vi "Engine Dynamics.vi"(6 "dt":sgl=1.0 format="%0.2f", 8 "phi":sgl, 9 "Impeller Torque (N-m)":sgl, 10 "Spark Advance (deg BTDC)":sgl, 11 "Throttle Angle (deg)":sgl) -> (1 "Torque (N-m)":sgl, 2 "Engine Speed (rad/s)":sgl format="%0.2f", 3 "Manifold Pressure (bar)":sgl format="%0.2f")   [LabVIEW 2016, in "NI-PCG Vehicle Model.lvlib"]
uses:
  NI-PCG Vehicle Model.lvlib
  Globals/Parameters.vi
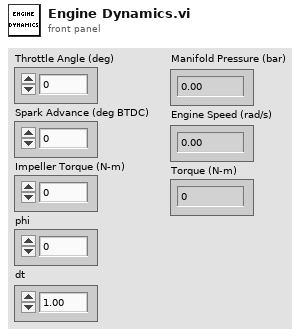
[diagram p1: front panel]
types:
  T1 = typedef "NI-PCG Vehicle Model.lvlib/Engine Parameters.ctl" = cluster{"Ambient Parameters":cluster{"Temperature (K)":sgl, "Pressure (Pa)":sgl}, "Air Parameters":cluster{"R (Ideal Gas Constant)":sgl, "Molecular Weight":sgl, "Cp (Specific Heat Constant)":sgl, "Density (kg/m^3)":sgl, "Stoichiometric A/F Ratio":sgl}, "Engine Geometry Parameters":cluster{"Cylinder Volume (l)":sgl, "J (Rotational Moment of Inertia)":sgl, "Minimuim Engine Speed":sgl, "Maximum Engine Speed":sgl, "Intake Manifold Volume (l)":sgl}, "Volumetric Efficiency Map":cluster{"MAP":sgl[], "RPM":sgl[], "Table":sgl[][]}, "Fuel LHV (J/kg)":sgl, "Combustion Efficiency Map":cluster{"Spark Timing (deg BTDC))":sgl[], "Engine Speed (RPM)":sgl[], "Combustion Efficiency":sgl[][]}, "Thermodynamic Efficiency":sgl}
  T2 = typedef "NI-PCG Vehicle Model.lvlib/Transmission Parameters.ctl" = cluster{"Final Drive Ratio":sgl, "Transmission Gear Ratios":cluster{"Gears":sgl[], "Gear Ratios":sgl[]}, "Torque Converter Map":cluster{"Speed Ratio":sgl[], "K Factor":sgl[], "Torque Ratio":sgl[]}, "Upshift Throttle":sgl[], "Downshift Throttle":sgl[], "Upshift Table":sgl[][], "Downshift Table":sgl[][], "Wait Time":u8}
  T3 = typedef "NI-PCG Vehicle Model.lvlib/Vehicle Parameters.ctl" = cluster{"Vehicle Mass (kg)":sgl, "Vehicle Cd":sgl, "Vehicle Frontal Area (m^2)":sgl, "Wheel Radius (m)":sgl, "Wheel Rolling Resistance":sgl}
  T4 = cluster{"Engine Parameters":T1, "Transmission Parameters":T2, "Vehicle Parameters":T3}
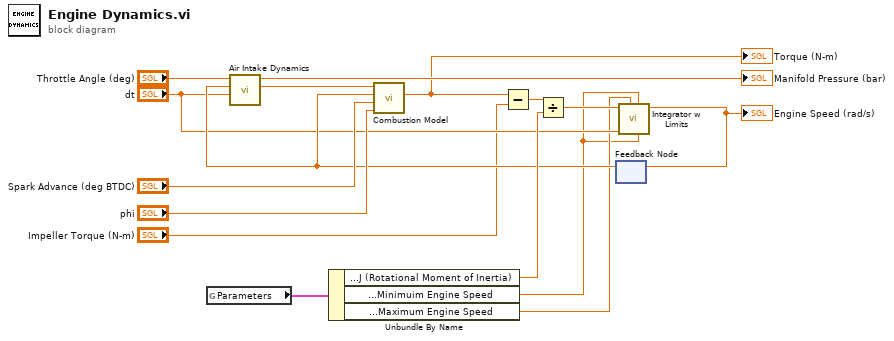
[diagram p0: block diagram]
diagram:
  n1 = global read "Parameters.vi" "Parameters"() -> (w7:T4)
  n2 = Unbundle By Name(w7) -> ("Engine Parameters.Engine Geometry Parameters.J (Rotational Moment of Inertia)"=w10:sgl, "Engine Parameters.Engine Geometry Parameters.Minimuim Engine Speed"=w1:sgl, "Engine Parameters.Engine Geometry Parameters.Maximum Engine Speed"=w4:sgl)
  n3 = feedback #1() -> (w9:sgl)  [unwired: 1 in]
  n4 = call "Air Intake Dynamics.vi"("dt"="dt", "Engine Speed (rad/s)"=w9, "Throttle Angle (deg)"="Throttle Angle (deg)") -> ("Air Mass/Cycle (g)"=w16:sgl, "Manifold Pressure (bar)"=→"Manifold Pressure (bar)":sgl)  [unwired: 7 in]
  n5 = call "Combustion Model.vi"("phi"="phi", "Spark Advance (deg BTDC)"="Spark Advance (deg BTDC)", "Engine Speed (rad/s)"=w9, "Air Charge (g)"=w16) -> ("Torque (N-m)"=w3:sgl)  [unwired: 7 in]
  "Torque (N-m)" <- w3
  n6 = Subtract(x=w3, y="Impeller Torque (N-m)") -> (x-y=w11:sgl)
  n7 = Divide(x=w11, y=w10) -> (x/y=w6:sgl)
  n8 = call "Integrator w Limits.vi"("Initial Condition"=w1, "lower limit"=w1, "upper limit"=w4, "dt [s]"="dt", "x"=w6) -> ("Result"=w8:sgl)  [unwired: 6 in]
  "Engine Speed (rad/s)" <- w8
  n9 = feedback-in #1(w8) -> ()
